vi "Close Device Core.vi"(8 "error in (no error)":errorcluster, 11 "BNT_DAQmx-MCSV-DOPWM in":refnum<class "BNT_DAQmx-MCSV-DOPWM.lvclass">) -> (0 "error out":errorcluster, 3 "BNT_DAQmx-MCSV-DOPWM out":refnum<class "BNT_DAQmx-MCSV-DOPWM.lvclass">)   [LabVIEW 2020, in "BNT_DAQmx.lvlib" / "BNT_DAQmx-MCSV-DOPWM.lvclass"]
doc: "Close device driver connection."
uses:
  BNT_DAQmx-MCSV-DOPWM.lvclass
  C:/Users/holge/Documents/LVP/BNT/PGC/Packages/BNT_DAQmx/BNT_DAQmx-MCSV/BNT_DAQmx-MCSV.lvclass
  BNT_DAQmx-MCSV/BNT_DAQmx-MCSV.lvclass/BNT_DAQmx-MCSV.ctl
  BNT_DAQmx-MCSV/BNT_DAQmx-MCSV.lvclass
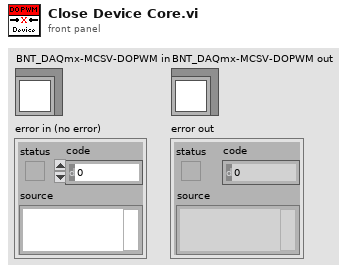
[diagram p1: front panel]
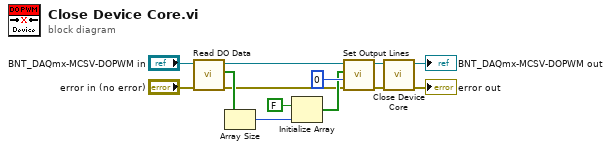
[diagram p0: block diagram]
diagram:
  n1 = call "Read DO Data.vi"("error in (no error)"="error in (no error)", "BNT_DAQmx-MCSV in"="BNT_DAQmx-MCSV-DOPWM in") -> ("error out"=w3:errorcluster, "DO Data"=w5:bool[], "BNT_DAQmx-MCSV out"=w1:refnum<class "BNT_DAQmx-MCSV-DOPWM.lvclass">)  [unwired: 7 in]
  n2 = Array Size(array=w5) -> (size(s)=w9:i32)
  n3 = Initialize Array(FALSE, w9) -> (w10:bool[])
  n4 = call "Set Output Lines.vi"("Error In"=w3, "Start Index"=0, "DO Lines"=w10, "BNT_DAQmx-MCSV in"=w1) -> ("Error Out"=w7:errorcluster, "BNT_DAQmx-MCSV out"=w6:refnum<class "BNT_DAQmx-MCSV-DOPWM.lvclass">)  [unwired: 6 in]
  n5 = call-parent "Close Device Core.vi"("error in (no error)"=w7, "BNT_DAQmx-MCSV in"=w6) -> ("error out"=→"error out":errorcluster, "BNT_DAQmx-MCSV out"=→"BNT_DAQmx-MCSV-DOPWM out":refnum<class "BNT_DAQmx-MCSV-DOPWM.lvclass">)  [unwired: 8 in]
